vi "Teleop.vi"(10 "Match Info":T2={"Autonomous Elapsed Seconds"=0.0, "TeleOp Elapsed Seconds"=0.0, "Disabled Elapsed Seconds"=0.0, "Visited Autonomous"=FALSE, "Visited TeleOp"=FALSE, "Visited Disabled"=FALSE, "Autonomous Settings"={"Autonomous Style"=enum."Independent", "VI Refnum"=refnum}}, 11 "Call Context":T3) -> ()   [LabVIEW 2020]
doc: "This VI is called for each TeleOp packet received from the DS where the robot is not disabled. It is often used to read from the joysticks and update I/O or to update setpoints for timed control loops. It should complete and return within 20 milliseconds or it may miss DS packets."
uses:
  <vilib>/Rock Robotics/WPI/DriverStation/WPI_DriverStationDerivedRobotMode.ctl
  <vilib>/Rock Robotics/WPI/DriverStation/WPI_DriverStationMatch Info.ctl
  <vilib>/Rock Robotics/Network Tables/NT Read Boolean.vi
  <vilib>/Rock Robotics/WPI/Utilities/WPI_GetSetVariantRefNum.vi
  <vilib>/Rock Robotics/Network Tables/NT Read Number.vi
panel:
  out "sensor Position":dbl
  out "Heading":dbl
  out "Pitch":dbl
  out "Roll":dbl
  out "Yaw":dbl
  out "Raw Values":T1 {"Accel X" format="%.8f"; "Accel Y" format="%.8f"; "Accel Z" format="%.8f"; "Gyro X" format="%.8f"; "Gyro Y" format="%.8f"; "Gyro Z" format="%.8f"; "Mag X" format="%.8f"; "Mag Y" format="%.8f"; "Mag Z" format="%.8f"}
  out "Gripper Command":dbl
  out "arm error out":errorcluster
  out "Sample Slider 0":dbl(slide) scale=0.0..5.0
  out "Sample Boolean 1":bool
  out "Sample Boolean 0":bool
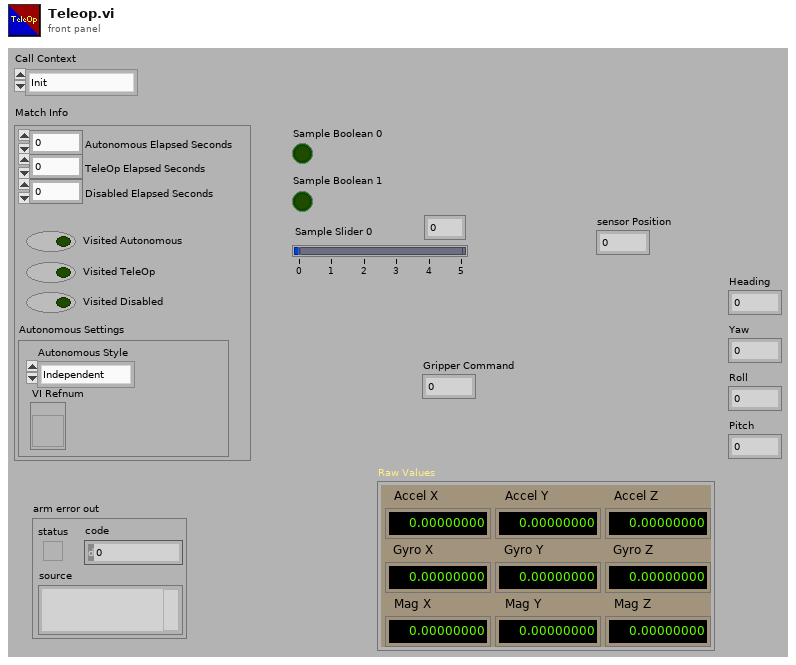
[diagram p1: front panel]
types:
  T1 = cluster{"Accel X":dbl, "Accel Y":dbl, "Accel Z":dbl, "Gyro X":dbl, "Gyro Y":dbl, "Gyro Z":dbl, "Mag X":dbl, "Mag Y":dbl, "Mag Z":dbl}
  T2 = typedef "WPI_DriverStationMatch Info.ctl" = cluster{"Autonomous Elapsed Seconds":dbl, "TeleOp Elapsed Seconds":dbl, "Disabled Elapsed Seconds":dbl, "Visited Autonomous":bool, "Visited TeleOp":bool, "Visited Disabled":bool, "Autonomous Settings":cluster{"Autonomous Style":enum16{"Iterative", "Independent"}, "VI Refnum":refnum<vi>}}
  T3 = typedef "WPI_DriverStationDerivedRobotMode.ctl" = enum16{"Init", "Execute", "Stop"}
  T4 = typedef "WPI_JoystickDevRef.ctl" = cluster{"Device":T5}
  T5 = typedef "WPI_JoystickDeviceEnum.ctl" = enum16{"USB 0", "USB 1", "USB 2", "USB 3", "USB 4", "USB 5"}
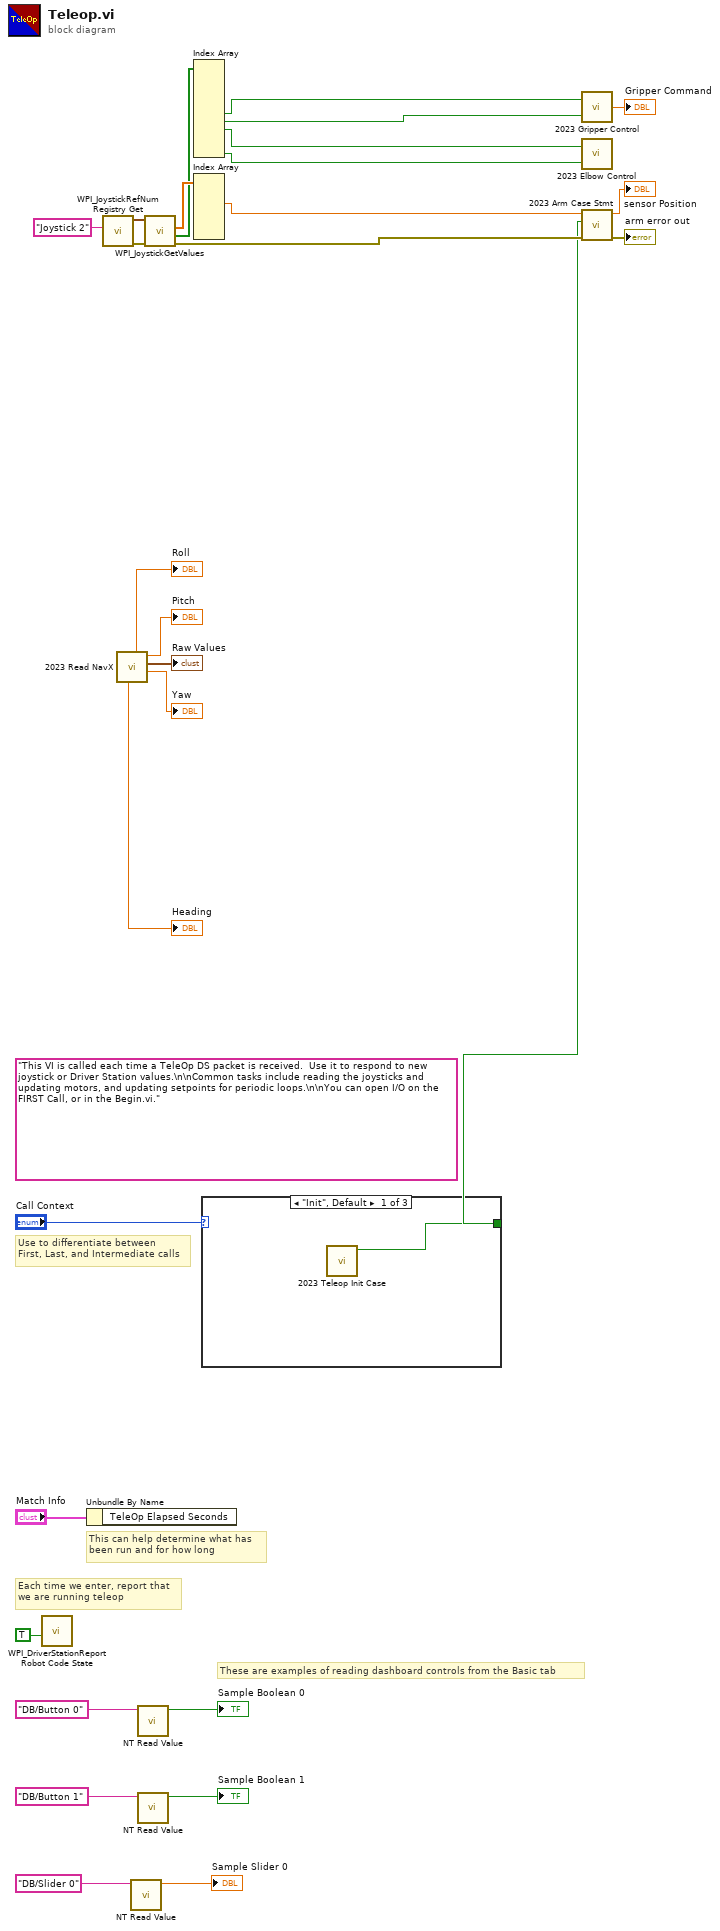
[diagram p0: block diagram]
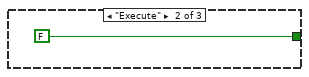
[diagram p2: hidden frame]
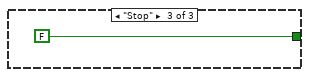
[diagram p3: hidden frame]
diagram:
  (unwired) "This VI is called each time a TeleOp DS packet is received.  Use it to respond to new joystick or Driver Station values.\n\nCommon tasks include reading the joysticks and updating motors, and updating setpoints for periodic loops.\n\nYou can open I/O on the FIRST Call, or in the Begin.vi."
  # "These are examples of reading dashboard controls from the Basic tab"
  # "Each time we enter, report that\nwe are running teleop"
  # "Use to differentiate between\nFirst, Last, and Intermediate calls"
  # "This can help determine what has\nbeen run and for how long"
  n1 = call <vilib>:"WPI_DriverStationReport Robot Code State.vi"("TeleOp"=TRUE ("Autonomous")) -> ()  [unwired: 10 in, 1 out]
  n2 = Unbundle By Name("Match Info") -> ()  [unwired: 1 out]
  n3 = call <vilib>:"WPI_JoystickRefNum Registry Get.vi"("refnum name"="Joystick 2") -> ("error out"=w20:errorcluster, "JoystickDevRef"=w19:T4)  [unwired: 1 in, 8 out]
  n4 = call "2023 Read NavX.vi"() -> ("Yaw"=→"Yaw":dbl, "Raw Values"=→"Raw Values":T1, "Pitch"=→"Pitch":dbl, "Roll"=→"Roll":dbl, "Heading"=→"Heading":dbl)  [unwired: 7 in]
  n5 = call-poly <vilib>:"NT Read Value.vi"("name"="DB/Slider 0" ("refnum name")) -> ("value"=→"Sample Slider 0":dbl)  [unwired: 8 in, 2 out]
  n6 = call-poly <vilib>:"NT Read Value.vi"("name"="DB/Button 0" ("refnum name")) -> ("value"=→"Sample Boolean 0":bool)  [unwired: 8 in, 2 out]
  n7 = call-poly <vilib>:"NT Read Value.vi"("name"="DB/Button 1" ("refnum name")) -> ("value"=→"Sample Boolean 1":bool)  [unwired: 8 in, 2 out]
  n8 = call <vilib>:"WPI_JoystickGetValues.vi"("error in (no error)"=w20, "JoystickDevRef"=w19) -> ("error out"=w11:errorcluster, "Buttons"=w17:bool[], "Axes"=w21:dbl[])  [unwired: 5 in, 2 out]
  n9 = Index Array(array=w17) -> (element #5=w15:bool, element #6=w16:bool, element #7=w10:bool, element #10=w9:bool)  [unwired: 10 in, 6 out]
  n10 = Index Array(array=w21) -> (element #2=w12:dbl)  [unwired: 6 in, 5 out]
  n11 = case shown="\"Init\", Default" "Call Context" {
    tunnel: [w30 FALSE FALSE] -> w7
    frame "Init", Default {
      n12 = call "2023 Teleop Init Case.vi"() -> ("Boolean"=w30:bool)  [unwired: 11 in]
    }
    frame "Execute" {
    }
    frame "Stop" {
    }
  }
  n13 = call "2023 Gripper Control.vi"("Button 6"=w16, "Button 5"=w15) -> ("Numeric"=→"Gripper Command":dbl)
  n14 = call "2023 Elbow Control.vi"("Button 6"=w9, "Button 5"=w10) -> ()  [unwired: 1 out]
  n15 = call "2023 Arm Case Stmt.vi"("error in (no error)"=w11, "Boolean"=w7, "upper limit"=w12) -> ("error out"=→"arm error out":errorcluster, "Sensor Position"=→"sensor Position":dbl)  [unwired: 7 in]
